vi "3-4.vi"() -> ()   [LabVIEW 2015]
panel:
  out "Cluster 2":cluster{"Name":string, "Age":dbl, "Age":bool}
  out "Cluster 1":cluster{"Name":string, "Age":dbl, "Sex":bool}
  in  "Sex":bool
  in  "Name":string
  in  "Age":dbl
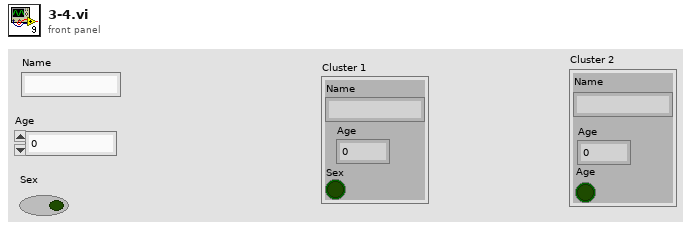
[diagram p1: front panel]
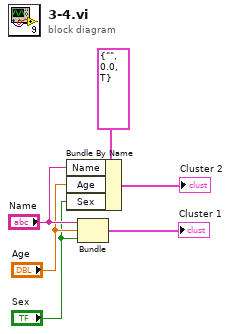
[diagram p0: block diagram]
diagram:
  n1 = Bundle By Name(cluster=cluster{"Name":string, "Age":dbl, "Sex":bool} {"Name"="", "Age"=0.0, "Sex"=TRUE} ("input cluster"), "Name"="Name", "Age"="Age", "Sex"="Sex") -> (→"Cluster 2":cluster{"Name":string, "Age":dbl, "Sex":bool})
  n2 = Bundle("Name"="Name", "Age"="Age", "Sex"="Sex") -> (→"Cluster 1":cluster{"Name":string, "Age":dbl, "Sex":bool})  [unwired: 1 in]
